vi "Added Value.vi"(8 "error in (no error)":errorcluster, 10 "Element in":refnum<class "Abs_Value.lvclass">, 11 "Fault-Injection_Boolean in":refnum<class "Fault-Injection_I8.lvclass">) -> (0 "error out":errorcluster, 3 "Fault-Injection_Boolean out":refnum<class "Fault-Injection_I8.lvclass">)   [LabVIEW 2021, in "Fault-Injection_I8.lvclass"]
uses:
  Fault-Injection_I8.lvclass
  <vilib>/TSA/Abstract Data Classes/Abs_Types/Value/Abs_Value.lvclass
  Fault-Injection_I8.lvclass/Fault-Injection_I8.ctl
  Support/Abs Class Type.ctl
  <vilib>/TSA/Abstract Data Classes/Abs_Types/I8 Integer/Abs_I8 Integer.lvclass
  Support/DVR Type.ctl
  Support/Value Type.ctl
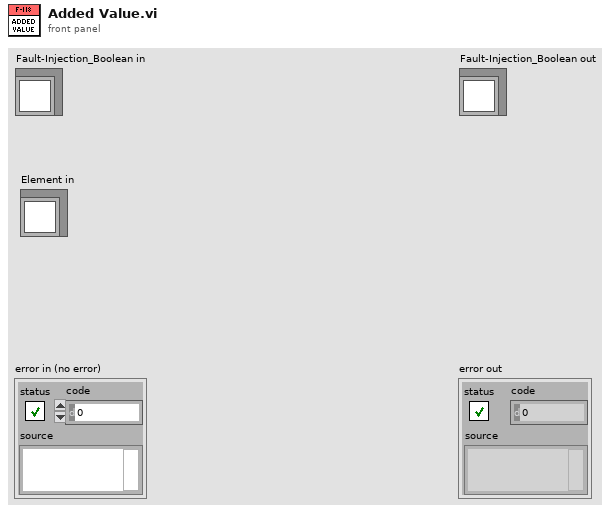
[diagram p1: front panel]
types:
  T1 = typedef "Fault-Injection_I8.lvclass/Abs Class Type.ctl" = refnum<class "Abs_I8 Integer.lvclass">
  T2 = typedef "Fault-Injection_I8.lvclass/DVR Type.ctl" = cluster{"Enable":bool, "Injected Value":T3, "Value":T1}
  T3 = typedef "Fault-Injection_I8.lvclass/Value Type.ctl" = i8
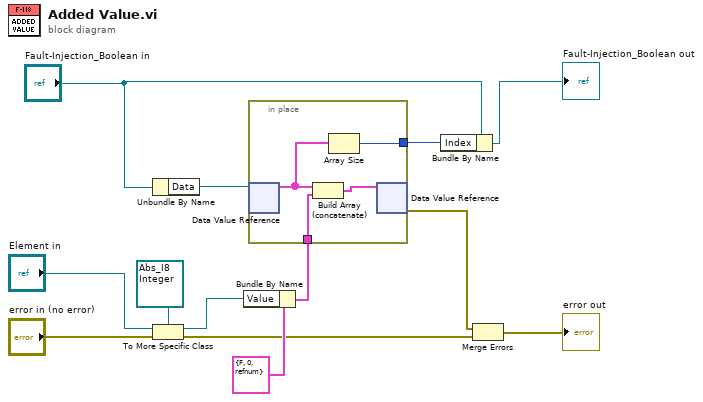
[diagram p0: block diagram]
diagram:
  n1 = Unbundle By Name("Fault-Injection_Boolean in") -> ("Data"=w13:refnum<data-value>)
  n2 = To More Specific Class(target class=T1 refnum ("Boolean in"), reference="Element in", error in="error in (no error)") -> (specific class reference=w10:T1, error out=w3:errorcluster)
  n3 = Bundle By Name(cluster=T2 {"Enable"=FALSE, "Injected Value"=0, "Value"=refnum} ("Cluster"), "Value"=w10) -> (w8:T2)
  n4 = in-place {
    in-place-border: w8 -> [w16]
    in-place-border: [w14] -> w6
    n5 = in-place-dvr #1(w13) -> (w15:T2[])  [unwired: 1 out]
    n6 = Build Array (concatenate)(w15, w16) -> (w17:T2[])
    n7 = Array Size(array=w15) -> (size(s)=w14:i32)
    n8 = in-place-dvr #1(w17) -> (w2:errorcluster)  [unwired: 1 out]
  }
  n9 = Bundle By Name(cluster="Fault-Injection_Boolean in", "Index"=w6) -> (→"Fault-Injection_Boolean out":refnum<class "Fault-Injection_I8.lvclass">)
  n10 = Merge Errors(w2, w3) -> (→"error out":errorcluster)
